vi "development sandbox 1.vi"() -> ()   [LabVIEW 2016]
uses:
  Suggestions IO/Static Listbox IO/Static Listbox IO.lvclass
  E:/Repository/LabVIEW Intellisense Script Editor/source/Suggestions IO/base/SuggestionIObase.lvclass
  Suggestions IO/Static Listbox IO/Static Listbox IO.lvclass/Static Listbox IO.ctl
  Suggestions IO/Static Listbox IO/Properties/Write Suggestion Listbox.vi
  String IntelliSense library/Polymorphic APIs/Instantiate IntelliSenseString.vi
  String IntelliSense library/Polymorphic APIs/Destroy All.vi
  String IntelliSense library/StringIntelliSense.lvlib
panel:
  in  "Suggestions":i32(listbox)
  in  "Script":string
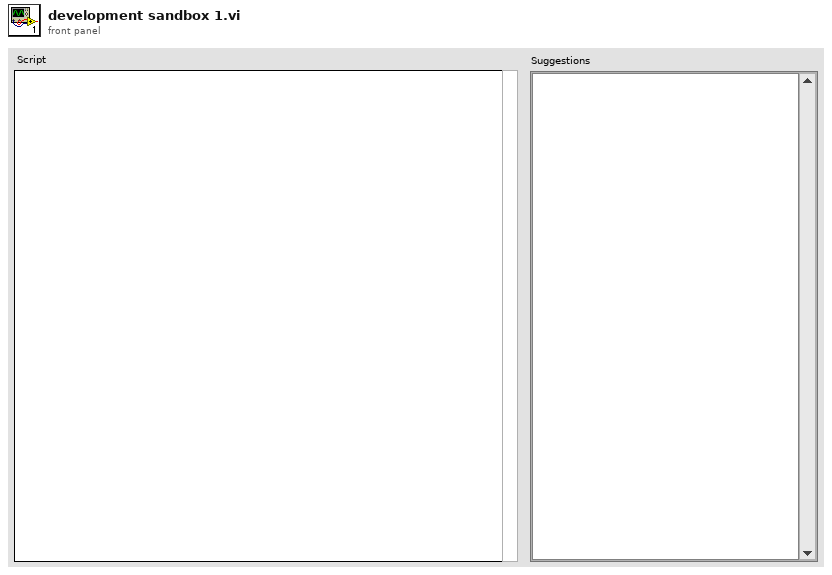
[diagram p1: front panel]
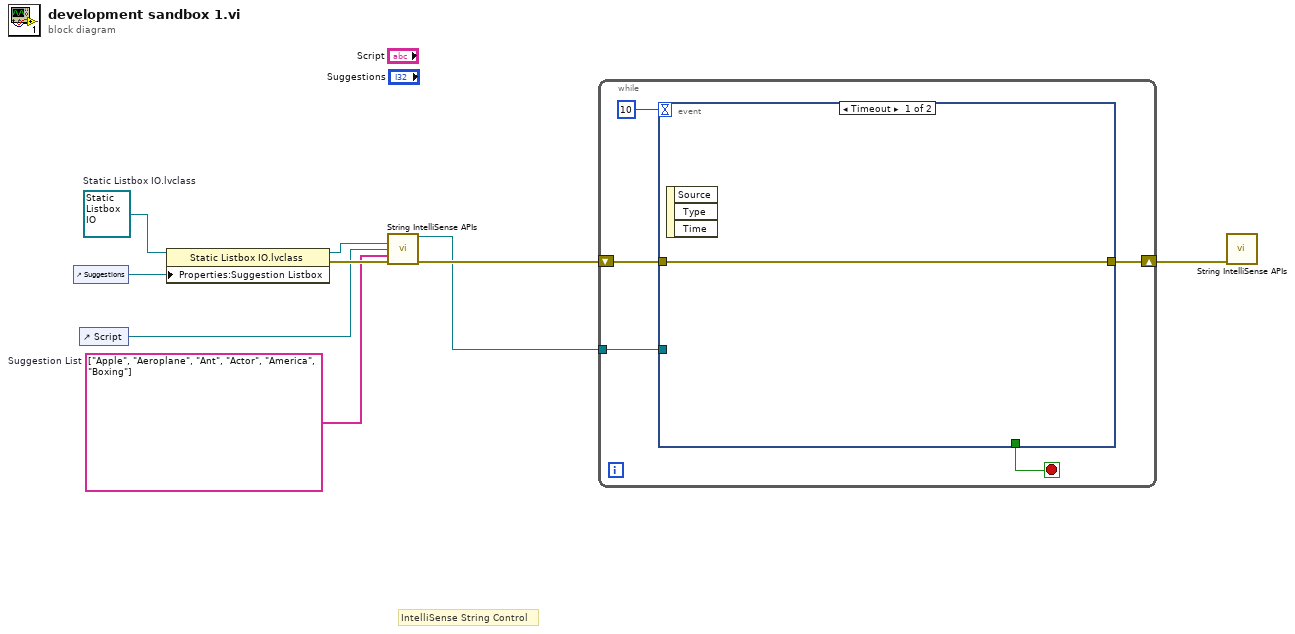
[diagram p0: block diagram]
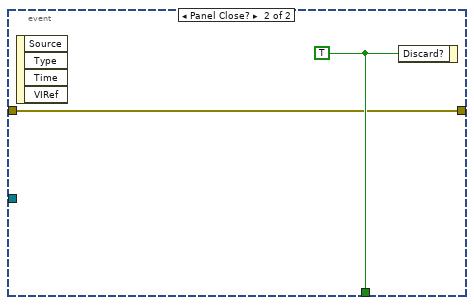
[diagram p2: hidden frame]
diagram:
  w2 = string[] ["Apple", "Aeroplane", "Ant", "Actor", "America", "Boxing"]  # Suggestion List
  w7 = refnum<class "Static Listbox IO.lvclass"> refnum  # Static Listbox IO.lvclass
  # "IntelliSense String Control"
  n1 = control-ref of="Suggestions"() -> (w6:refnum<vi>)
  n2 = control-ref of="Script"() -> (w4:refnum<vi>)
  n3 = property class="Static Listbox IO.lvclass"(reference=w7, "Properties:Suggestion Listbox"=w6) -> (reference out=w3:refnum<class "Static Listbox IO.lvclass">, error out=w5:errorcluster)  [unwired: 1 in]
  n4 = call-poly "String IntelliSense APIs.vi"("Suggestion IO in"=w3, "Str Ctl Refnum"=w4, "Str ctrl Suggestion"=w2, "error in (no error)"=w5) -> ("IntelliSense String"=w1:refnum<class "IntelliSenseStringControl.lvclass">, "error out"=w9:errorcluster)  [unwired: 10 in]
  n5 = while {
    shift-right: [w12] -> w8
    shift-left: w9 -> [w13]
    tunnel: w1 -> [w10]
    stop <- w11 stop-if-true
    n6 = event shown="[0] Timeout" {
      selector: _ -> [_ _]
      dyn-events: _ -> [_ _]
      timeout: 10 -> [_ _]
      tunnel: w13 -> [w15 w16]
      tunnel: [w15 w16] -> w12
      tunnel: [_ w17] -> w11
      tunnel: w10 -> [_ _]
      event Timeout {
        n7 = event-data() -> ()  [unwired: 1 in, 3 out]
      }
      event Panel Close? {
        w17 = TRUE ("Discard?")
        n8 = event-data() -> ()  [unwired: 1 in, 4 out]
        n9 = event-data("Discard?"=w17) -> ()  [unwired: 1 in, 1 out]
      }
    }
  }
  n10 = call-poly "String IntelliSense APIs.vi"("error in (no error)"=w8) -> ()  [unwired: 14 in, 1 out]
